vi "start kill devs.vi"(5 "All Devices Core Info":string[][](array[string]), 6 "time between commands (ms)":u32, 7 "Local Port":u16, 8 "error in (no error)":errorcluster, 9 "Device Names for scan data":string[](array[string]), 10 "class []":string[](array[string]), 11 "Device Names for scan data 2":string[](array[string])) -> (0 "error out":errorcluster, 3 "IP Addresses":string[](array[string]))   [LabVIEW 2020]
uses:
  <userlib>/_OpenG.lib/array/array.llb/Sort 2D Array (String)__ogtk.vi
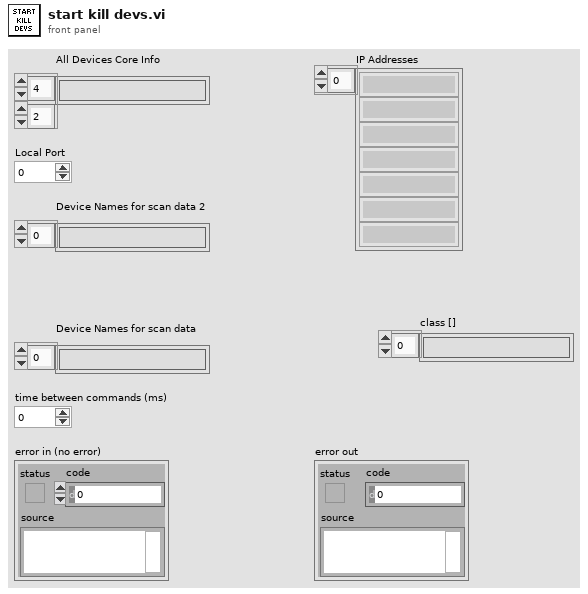
[diagram p1: front panel]
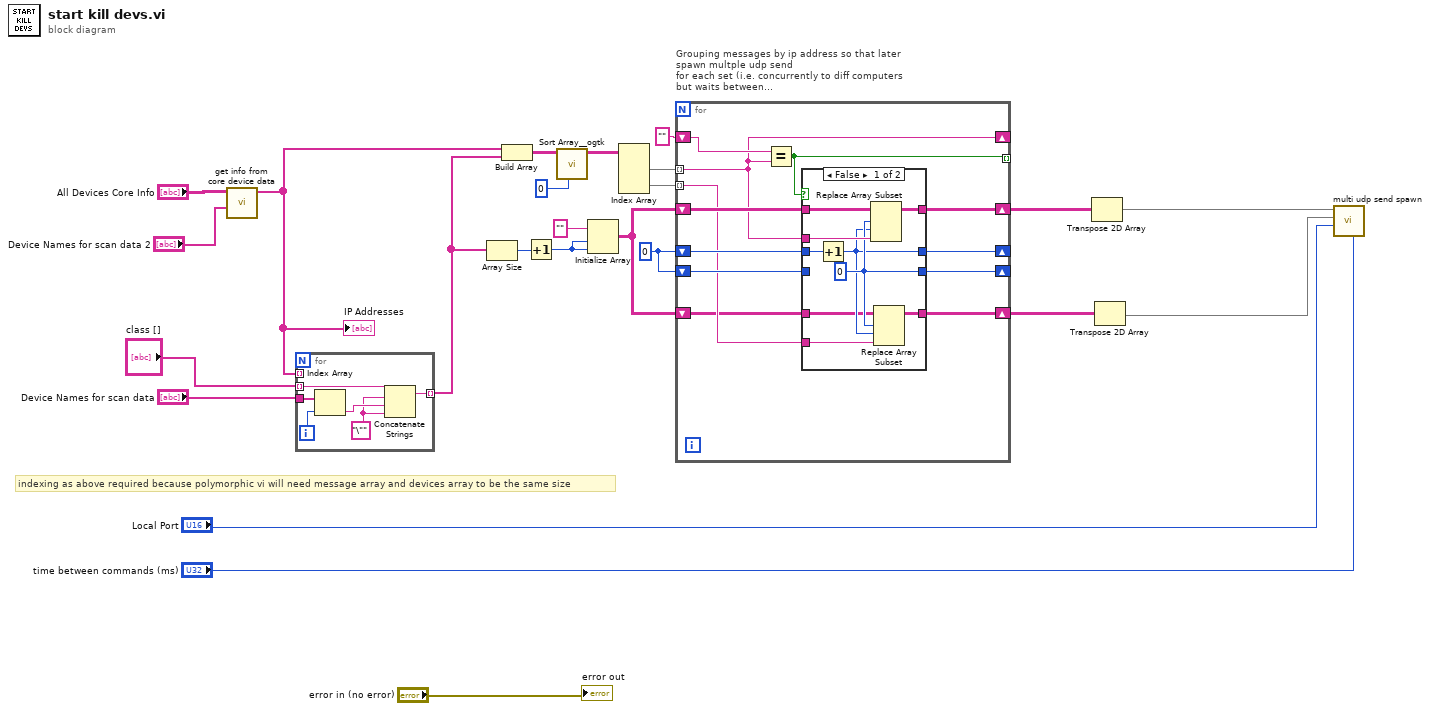
[diagram p0: block diagram]
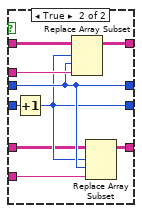
[diagram p2: hidden frame]
diagram:
  w11 = 0
  # "indexing as above required because polymorphic vi will need message array and devices array to be the same size"
  n1 = call "get info from core device data.vi"("devices to get data from"="Device Names for scan data 2", "All Devices Core Info"="All Devices Core Info") -> ("IP Addresses"=w1:string[])  [unwired: 1 in, 4 out]
  "IP Addresses" <- w1
  n2 = for {
    tunnel: "class []" -> [w30] mode=indexing
    tunnel: "Device Names for scan data" -> [w27]
    tunnel: [w29] -> w13 mode=indexing
    tunnel: w1 -> [_] mode=indexing
    i -> [w28]
    w25 = "\"" ("string")
    n3 = Index Array(array=w27, index=w28) -> (element=w26:string)
    n4 = Concatenate Strings(w30, w25, w26, w25) -> (w29:string)
  }
  n5 = Array Size(array=w13) -> (size(s)=w14:i32)
  n6 = Build Array(w1, w13) -> (w6:string[][])
  n7 = Increment(x=w14) -> (x+1=w22:i32)
  n8 = call-poly <userlib>:"Sort Array__ogtk.vi"("Column/Row to Sort By"=u32 0, "Array in"=w6) -> ("Sorted Array out"=w9:string[][])  [unwired: 6 in, 3 out]
  n9 = Initialize Array("" ("String"), w22, w22) -> (w15:string[][])
  n10 = Index Array(array=w9) -> (element #1=w10:string[], element #2=w16:string[])  [unwired: 4 in]
  n11 = for "Grouping messages by ip address so that later spawn multple udp send\nfor each set (i.e. concurrently to diff computers but waits between\neach device start on a given computer)" {
    shift-right: [w39] -> _
    shift-left: "" ("String") -> [w42]
    tunnel: [w41] -> _ mode=indexing
    tunnel: w10 -> [w39] mode=indexing
    shift-right: [w38] -> w17
    shift-left: w15 -> [w40]
    shift-right: [w36] -> _
    shift-left: w11 -> [w37]
    shift-right: [w34] -> _
    shift-left: w11 -> [w35]
    shift-right: [w31] -> w18
    shift-left: w15 -> [w32]
    tunnel: w16 -> [w33] mode=indexing
    n12 = Equal?(x=w42, y=w39) -> (x = y?=w41:bool)
    n13 = case shown="False" w41 {
      tunnel: w40 -> [w49 w59]
      tunnel: w39 -> [w48 w57]
      tunnel: [w50 w58] -> w38
      tunnel: w37 -> [w51 w56]
      tunnel: [w46 w56] -> w36
      tunnel: w35 -> [_ w60]
      tunnel: [w47 w55] -> w34
      tunnel: w33 -> [w45 w54]
      tunnel: w32 -> [w44 w53]
      tunnel: [w43 w52] -> w31
      frame False {
        w47 = 0
        n14 = Increment(x=w51) -> (x+1=w46:i32)
        n15 = Replace Array Subset(array=w49, new element=w48, index (row)=w47, index (col)=w46) -> (w50:string[][])
        n16 = Replace Array Subset(array=w44, new element=w45, index (row)=w47, index (col)=w46) -> (w43:string[][])
      }
      frame True {
        n17 = Increment(x=w60) -> (x+1=w55:i32)
        n18 = Replace Array Subset(array=w59, new element=w57, index (row)=w55, index (col)=w56) -> (w58:string[][])
        n19 = Replace Array Subset(array=w53, new element=w54, index (row)=w55, index (col)=w56) -> (w52:string[][])
      }
    }
  }
  n20 = Transpose 2D Array(2D array=w17) -> (transposed array=w19:string[][])
  n21 = Transpose 2D Array(2D array=w18) -> (transposed array=w20:string[][])
  n22 = call "multi udp send spawn.vi"("IP array"=w19, "Message array"=w20, "Local udp lv starter port"="Local Port", "time between commands (ms)"="time between commands (ms)") -> ()  [unwired: 4 in, 1 out]
  "error out" <- "error in (no error)"
